vi "Handle Vehicle out of Position.vi"(8 "error in (no error)":errorcluster, 10 "Vehicle out of Position":bool, 11 "Car Wash Model in":refnum<class "Car Wash Model.lvclass">) -> (0 "error out":errorcluster, 3 "Car Wash Model out":refnum<class "Car Wash Model.lvclass">)   [LabVIEW 2019, in "Car Wash Model.lvclass"]
uses:
  <vilib>/gpm_packages/@cs/Car-wash/Source/Car Wash Model/Car Wash Model/Car Wash Model.lvclass
  <vilib>/gpm_packages/@cs/Car-wash/Source/Car Wash Model/Car Wash Model/Car Wash Model.lvclass/Car Wash Model.ctl
  <vilib>/ActorFramework/Message Enqueuer/Message Enqueuer.lvclass/Message Enqueuer.ctl
  <vilib>/ActorFramework/Message Enqueuer/Enqueue.vi
  <vilib>/gpm_packages/@cs/Car-wash/Source/iProcess Model/iProcess Model Messages/Resume Process Msg/Resume Process Msg.lvclass
  C:/Program Files/National Instruments/LabVIEW 2019/vi.lib/ActorFramework/Message/Message.lvclass
  <vilib>/ActorFramework/Message Priority Queue/Priority Enqueue.vi
  <vilib>/gpm_packages/@cs/Car-wash/Source/iProcess Model/iProcess Model Messages/Pause Process Msg/Pause Process Msg.lvclass
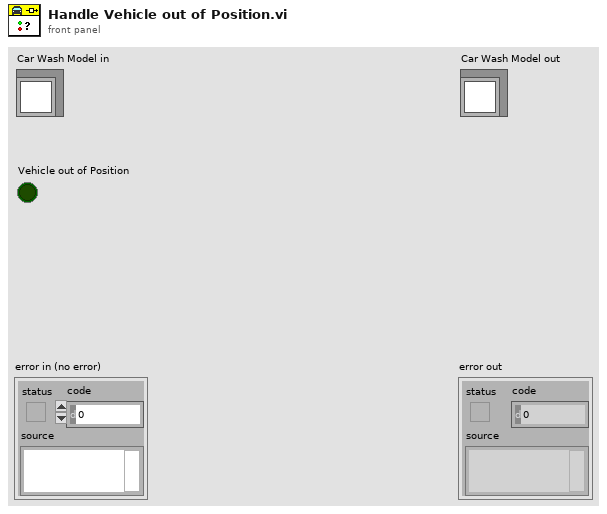
[diagram p1: front panel]
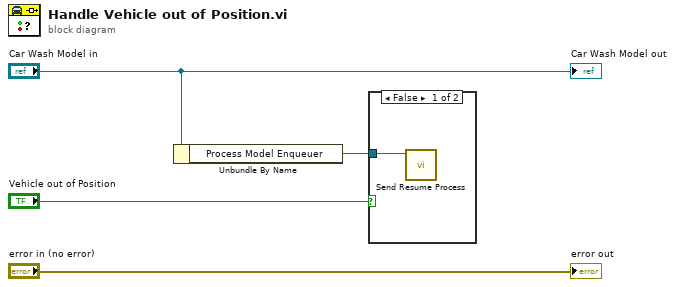
[diagram p0: block diagram]
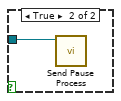
[diagram p2: hidden frame]
diagram:
  n1 = Unbundle By Name("Car Wash Model in") -> ("Process Model Enqueuer"=w1:refnum<class "Message Enqueuer.lvclass">)
  n2 = case shown="False" "Vehicle out of Position" {
    tunnel: w1 -> [w5 w6]
    frame False {
      n3 = call <vilib>:"Send Resume Process.vi"("Message Enqueuer"=w5) -> ()  [unwired: 9 in, 2 out]
    }
    frame True {
      n4 = call <vilib>:"Send Pause Process.vi"("Message Enqueuer"=w6) -> ()  [unwired: 9 in, 2 out]
    }
  }
  "error out" <- "error in (no error)"
  "Car Wash Model out" <- "Car Wash Model in"
